vi "Get ObjData.vi"(8 "error in (no error)":errorcluster, 11 "Database in":refnum<class "Database.lvclass">) -> (0 "error out":errorcluster, 2 "ObjData":T1, 3 "Database out":refnum<class "Database.lvclass">)   [LabVIEW 2022 SP3, in "Database.lvclass"]
doc: "Developed by Kevin Thompson\nkevin@thompsonengineering.net\n\nCopyright 2018\nThompson Engineering, LLC"
uses:
  Database.lvclass
  DataTypes/ObjData--cluster.ctl
  DataTypes/Settings--cluster.ctl
  DataTypes/Public Events--cluster.ctl
  Common/Controls/TD Async CmdMsg EventData--cluster.ctl
  Common/Controls/TD Sync API Event Data.ctl
  Common/Controls/APIReturnCluster--Cluster.ctl
  Common/Controls/TD Sync API Task State.ctl
  DataTypes/Dependency--cluster.ctl
  DataTypes/Read Data--cluster.ctl
  Database.lvclass/Database.ctl
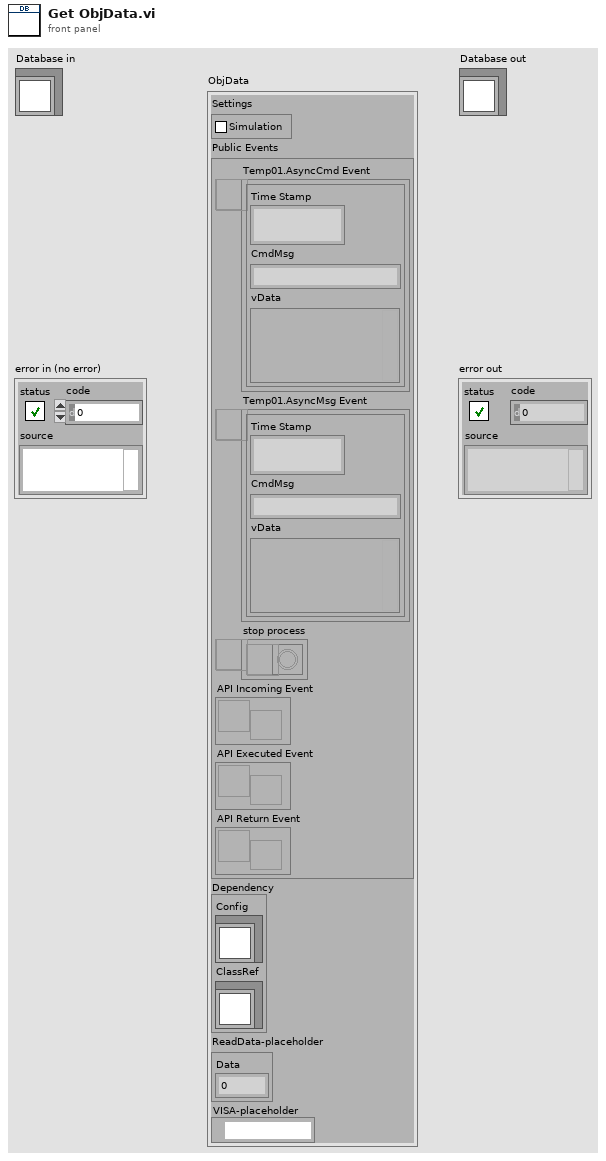
[diagram p1: front panel]
types:
  T1 = typedef "Database.lvclass/ObjData--cluster.ctl" = cluster{"Settings":T2, "Public Events":T3, "Dependency":T4, "ReadData-placeholder":T5, "VISA-placeholder":refnum<visa-resource-name>}
  T2 = typedef "Database.lvclass/Settings--cluster.ctl" = cluster{"Simulation":bool}
  T3 = typedef "Database.lvclass/Public Events--cluster.ctl" = cluster{"Temp01.AsyncCmd Event":refnum<user-event>, "Temp01.AsyncMsg Event":refnum<user-event>, "stop process":refnum<user-event>, "API Incoming Event":refnum<user-event>, "API Executed Event":refnum<user-event>, "API Return Event":refnum<user-event>}
  T4 = typedef "Database.lvclass/Dependency--cluster.ctl" = cluster{"Config":refnum<class>, "ClassRef":refnum<class>}
  T5 = typedef "Database.lvclass/Read Data--cluster.ctl" = cluster{"Data":dbl}
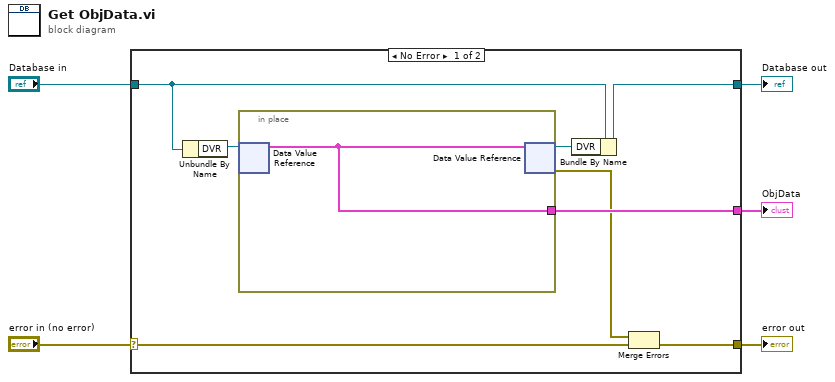
[diagram p0: block diagram]
diagram:
  n1 = case shown="No Error" "error in (no error)" {
    selector: "error in (no error)" -> [w13 w15]
    tunnel: [w7 w15] -> w4
    tunnel: [w9 w16] -> w2
    tunnel: "Database in" -> [w10 w16]
    tunnel: [w8 _] -> w1
    frame No Error {
      n2 = Unbundle By Name(w10) -> ("DVR"=w11:refnum<data-value>)
      n3 = in-place {
        in-place-border: [w14] -> w8
        n4 = in-place-dvr #1(w11) -> (w14:T1)  [unwired: 1 out]
        n5 = in-place-dvr #1(w14) -> (w12:refnum<data-value>, w6:errorcluster)
      }
      n6 = Bundle By Name(cluster=w10, "DVR"=w12) -> (w9:refnum<class "Database.lvclass">)
      n7 = Merge Errors(w6, w13) -> (w7:errorcluster)
    }
    frame Error {
    }
  }
  "error out" <- w4
  "Database out" <- w2
  "ObjData" <- w1
